vi "ZDataVIS_generate_format_paths.vi"(8 "error in (no error)":errorcluster, 10 "increment (T) or overwrite (F) folders":bool, 11 "File Information":T1={"File or folder path (input)"=path "G:/My Drive/ansom/Data/PPMS2/SA03008L.20190612/004_SG_IV_Testing", "output file description"="yonk"}) -> (0 "error out":errorcluster, 2 "Lockin Info DAT":path, 3 "Base processed output folder":path)   [LabVIEW 2016]
uses:
  <userlib>/_OpenG.lib/file/file.llb/Convert File Extension (Path)__ogtk.vi
  <vilib>/MakerHub/Toolbox/LMH-Toolbox.lvlib
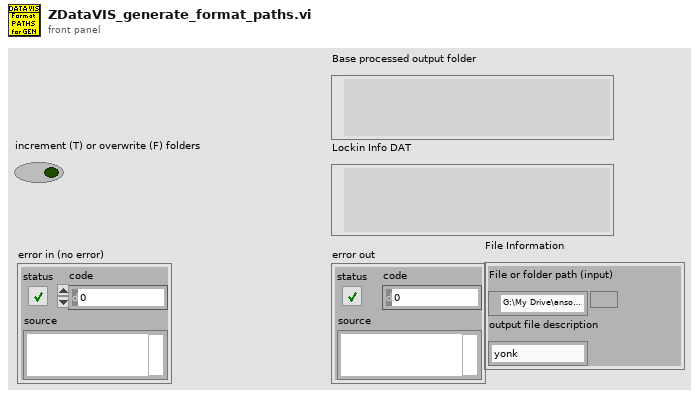
[diagram p1: front panel]
types:
  T1 = cluster{"File or folder path (input)":path, "output file description":string}
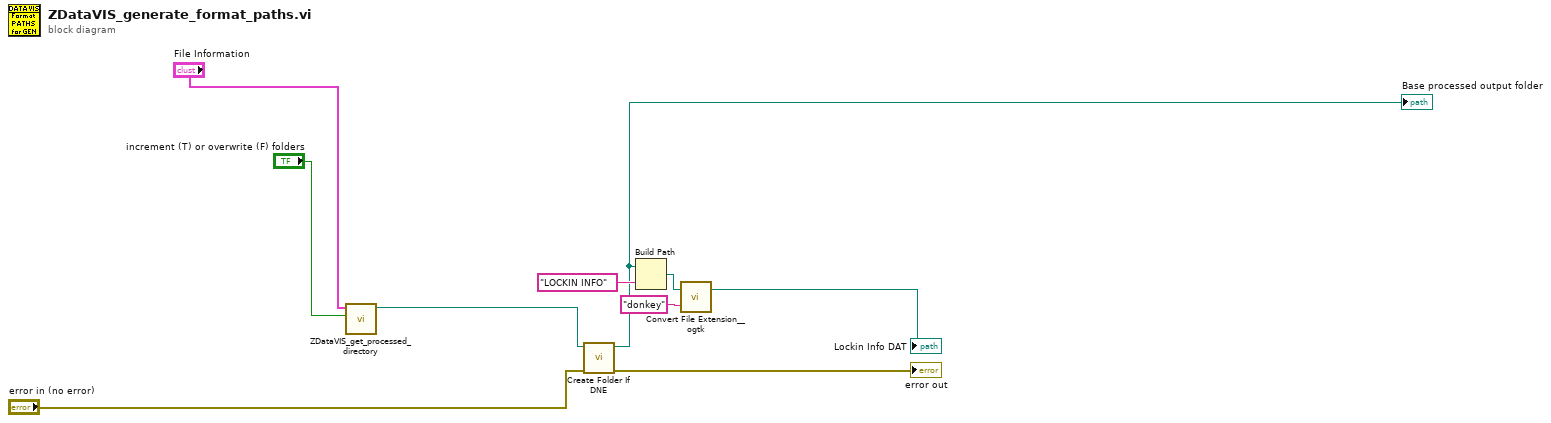
[diagram p0: block diagram]
diagram:
  n1 = call "ZDataVIS_get_processed_directory.vi"("increment (T) or overwrite (F) folders"="increment (T) or overwrite (F) folders", "File Information"="File Information") -> ("root processed directory"=w10:path)  [unwired: 9 in]
  n2 = call <vilib>:"Create Folder If DNE.vi"("Error In"="error in (no error)", "Folder Path"=w10) -> ("Error Out"=→"error out":errorcluster, "Dup Path"=w6:path)  [unwired: 8 in]
  "Base processed output folder" <- w6
  n3 = Build Path(base path=w6, name or relative path="LOCKIN INFO") -> (appended path=w4:path)
  n4 = call-poly <userlib>:"Convert File Extension__ogtk.vi"("new ending (none)"="donkey", "file name"=w4) -> ("new filename"=→"Lockin Info DAT":path)  [unwired: 1 out]
